vi "1.2.vi"() -> ()   [LabVIEW 2017]
panel:
  in  "停止":bool
  out "乘积结果":dbl
  in  "数值2":dbl
  in  "数值1":dbl
  in  "数值3":dbl
  in  "计算乘积":bool
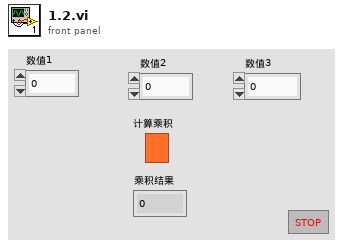
[diagram p1: front panel]
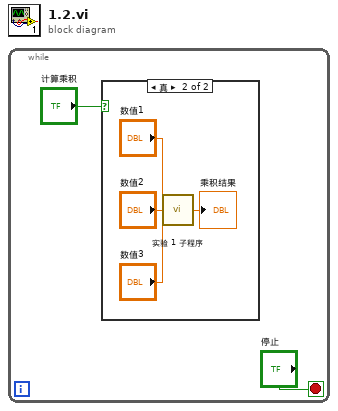
[diagram p0: block diagram]
diagram:
  n1 = while {
    stop <- "停止" stop-if-true
    n2 = case shown="真" "计算乘积" {
      frame False {
      }
      frame True {
        n3 = call "实验 1 子程序.vi"("数值 3"="数值3", "数值 2"="数值2", "数值1"="数值1") -> ("结果"=→"乘积结果":dbl)
      }
    }
  }
